vi "Project URL.vi"(10 "error in (no error)":errorcluster, 11 "DesignRequest":T1) -> (2 "error out":errorcluster, 3 "Project URL":string)   [LabVIEW 2012, in "Design Server.lvlib"]
uses:
  Design Server.lvlib
  Design Request.ctl
  Variable cluster.ctl
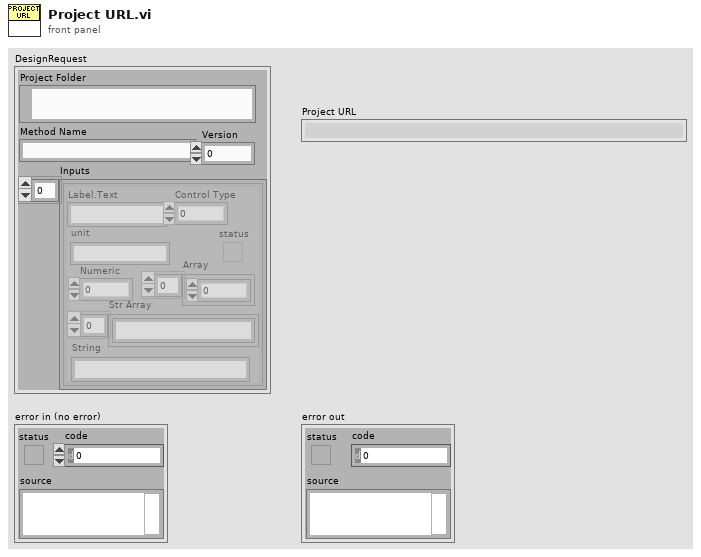
[diagram p1: front panel]
types:
  T1 = typedef "Design Server.lvlib/Design Request.ctl" = cluster{"Project Folder":path, "Method Name":string, "Inputs":T2, "Version":i32}
  T2 = typedef "Design Server.lvlib/Variable cluster.ctl" = cluster{"Label.Text":string, "Control Type":u32, "Numeric":dbl, "Array":dbl[], "status":bool, "Str Array":string[], "String":string, "unit":string}[]
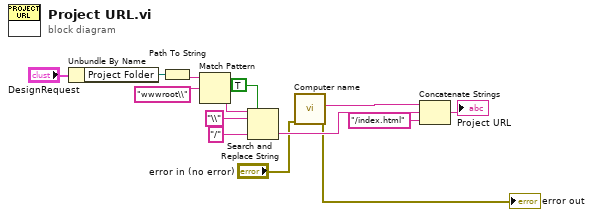
[diagram p0: block diagram]
diagram:
  n1 = Unbundle By Name("DesignRequest") -> ("Project Folder"=w8:path)
  n2 = Path To String(path=w8) -> (string=w6:string)
  n3 = Match Pattern(string=w6, regular expression="wwwroot\\") -> (after substring=w10:string)  [unwired: 1 in, 3 out]
  n4 = Search and Replace String(replace all?=TRUE ("replace all? (F)"), input string=w10, search string="\\", replace string="/" ("replace string (\"\")")) -> (result string=w11:string)  [unwired: 4 in, 3 out]
  n5 = call "Computer name.vi"("error in (no error)"="error in (no error)") -> ("error out"=→"error out":errorcluster, "Computer URL"=w14:string)  [unwired: 8 in, 1 out]
  n6 = Concatenate Strings(w14, w11, "/index.html" ("string")) -> (→"Project URL":string)
